vi "string to tag.vi"(8 "error in":errorcluster, 10 "tag string":string, 11 "tag descriptor in":refnum<class "tag descriptor.lvclass">) -> (0 "error out":errorcluster, 3 "tag descriptor out":refnum<class "tag descriptor.lvclass">)   [LabVIEW 2013, in "tag bus.lvlib" / "tag descriptor.lvclass"]
uses:
  tag descriptor.lvclass
  Data Type.ctl
  tag descriptor.lvclass/tag descriptor.ctl
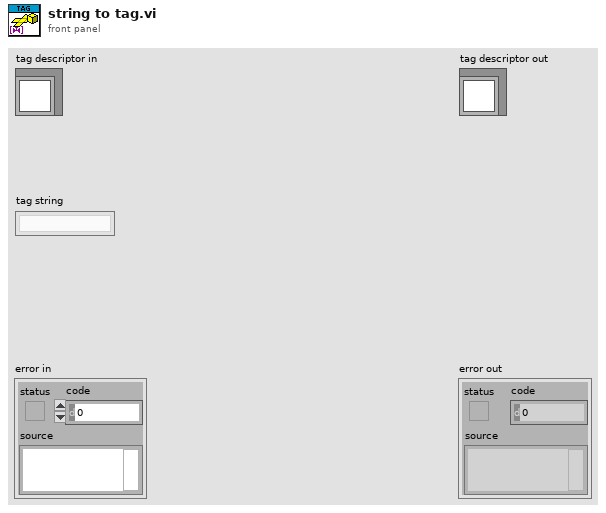
[diagram p1: front panel]
types:
  T1 = typedef "tag bus.lvlib/tag descriptor.lvclass/Data Type.ctl" = enum16{"Double", "Single", "I64", "I32", "I16", "I8", "U64", "U32", "U16", "U8", "Boolean", "String", "Array of Double", "Array of Single", "Array of I64", "Array of I32", "Array of I16", "Array of I8", "Array of U64", "Array of U32", "Array of U16", "Array of U8", "Array of Boolean", "Array of String"}
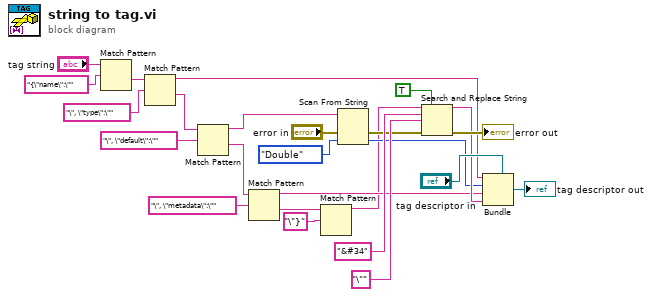
[diagram p0: block diagram]
diagram:
  n1 = Match Pattern(string="tag string", regular expression="{\"name\":\"") -> (after substring=w16:string)  [unwired: 1 in, 3 out]
  n2 = Match Pattern(string=w16, regular expression="\", \"type\":\"") -> (before substring=w14:string, after substring=w13:string)  [unwired: 1 in, 2 out]
  n3 = Match Pattern(string=w13, regular expression="\", \"default\":\"") -> (before substring=w9:string, after substring=w7:string)  [unwired: 1 in, 2 out]
  n4 = Match Pattern(string=w7, regular expression="\", \"metadata\":\"") -> (before substring=w5:string, after substring=w4:string)  [unwired: 1 in, 2 out]
  n5 = Match Pattern(string=w4, regular expression="\"}") -> (before substring=w1:string)  [unwired: 1 in, 3 out]
  n6 = Scan From String(input string=w9, error in="error in", default 1=Data_Type."Double" ("data type")) -> (error out=w2:errorcluster, output 1=w8:T1)  [unwired: 2 in, 2 out]
  n7 = Search and Replace String(replace all?=TRUE ("replace all? (F)"), input string=w1, search string="&#34" ("replace string (\"\")"), replace string="\"" ("search string"), error in=w2) -> (result string=w19:string, error out=→"error out":errorcluster)  [unwired: 3 in, 2 out]
  n8 = Bundle(cluster="tag descriptor in", w14, w8, w5, w19) -> (→"tag descriptor out":refnum<class "tag descriptor.lvclass">)
